vi "Replace Compiled Settings Cluster Constant.vi"(8 "error in":errorcluster, 10 "Compiled Settings ctl path":path, 11 "VI in":refnum<vi>) -> (0 "error out":errorcluster)   [LabVIEW 2026, in "NIVS_CDEW_MetaDataObj.lvclass"]
uses:
  NIVS_CDEW_MetaDataObj.lvclass
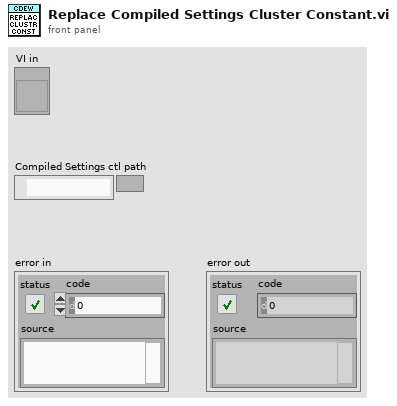
[diagram p1: front panel]
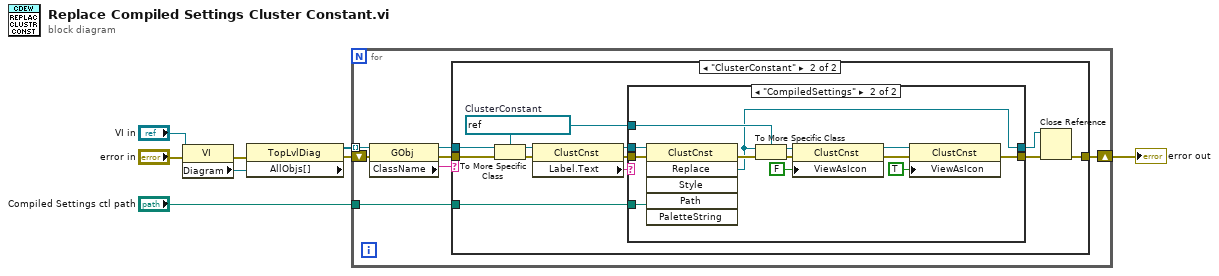
[diagram p0: block diagram]
diagram:
  n1 = property class="VI"(reference="VI in", error in="error in") -> (error out=w2:errorcluster, "Diagram"=w3:refnum<vi>)  [unwired: 1 out]
  n2 = property class="TopLvlDiag"(reference=w3, error in=w2) -> (error out=w6:errorcluster, "AllObjs[]"=w4:refnum<vi>[])  [unwired: 1 out]
  n3 = for {
    tunnel: w4 -> [w15] mode=indexing
    tunnel: "Compiled Settings ctl path" -> [w12]
    shift-right: [w11] -> w7
    shift-left: w6 -> [w10]
    n4 = property class="GObj"(reference=w15, error in=w10) -> (reference out=w13:refnum<vi>, error out=w14:errorcluster, "ClassName"=w9:string)
    n5 = case shown="\"ClusterConstant\"" w9 {
      tunnel: w14 -> [w16 w28]
      tunnel: w13 -> [_ w27]
      tunnel: w12 -> [_ w21]
      tunnel: [w16 w18] -> w11
      frame Default {
      }
      frame "ClusterConstant" {
        w17 = refnum<vi> refnum  # ClusterConstant
        n6 = To More Specific Class(target class=w17, reference=w27, error in=w28) -> (specific class reference=w25:refnum<vi>, error out=w26:errorcluster)
        n7 = property class="ClustCnst"(reference=w25, error in=w26) -> (reference out=w22:refnum<vi>, error out=w23:errorcluster, "Label.Text"=w24:string)
        n8 = case shown="\"CompiledSettings\"" w24 {
          tunnel: w23 -> [w29 w43]
          tunnel: w22 -> [w30 w42]
          tunnel: w21 -> [_ w41]
          tunnel: [w30 w31] -> w19
          tunnel: [w29 w33] -> w20
          tunnel: w17 -> [_ w40]
          frame Default {
          }
          frame "CompiledSettings" {
            n9 = invoke class="ClustCnst" method="Replace"(reference=w42, error in=w43, "Path"=w41) -> (error out=w34:errorcluster, "Replace"=w31:refnum<vi>)  [unwired: 3 in, 4 out]
            n10 = To More Specific Class(target class=w40, reference=w31, error in=w34) -> (specific class reference=w38:refnum<vi>, error out=w39:errorcluster)
            n11 = property class="ClustCnst"(reference=w38, error in=w39, "ViewAsIcon"=FALSE ("View As Icon")) -> (reference out=w35:refnum<vi>, error out=w36:errorcluster)
            n12 = property class="ClustCnst"(reference=w35, error in=w36, "ViewAsIcon"=TRUE ("View As Icon")) -> (error out=w33:errorcluster)  [unwired: 1 out]
          }
        }
        n13 = Close Reference(reference=w19, error in (no error)=w20) -> (error out=w18:errorcluster)
      }
    }
  }
  "error out" <- w7
